vi "cw_4_9.vi"() -> ()   [LabVIEW 2022 SP3]
panel:
  out "result string":string
  in  "String":string
  in  "Input":string
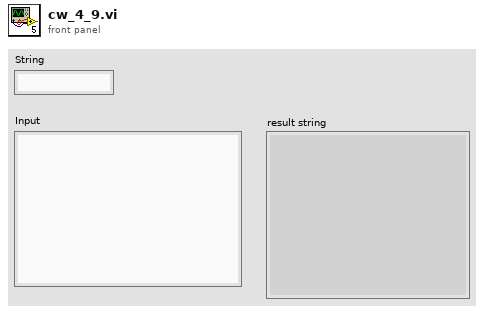
[diagram p1: front panel]
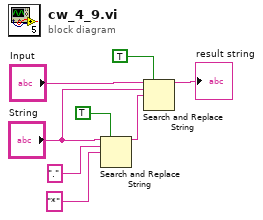
[diagram p0: block diagram]
diagram:
  n1 = Search and Replace String(replace all?=TRUE ("replace all? (F)"), input string="String", search string=".", replace string="*" ("replace string (\"\")")) -> (result string=w2:string)  [unwired: 4 in, 3 out]
  n2 = Search and Replace String(replace all?=TRUE ("replace all? (F)"), input string="Input", search string="String", replace string=w2) -> (result string=→"result string":string)  [unwired: 4 in, 3 out]
